vi "TestRUSH.vi"() -> ()   [LabVIEW 2012]
panel:
  out "Time in s":i32
  out "HavSetElevOut":i32
  in  "OutRoll":bool
  in  "Inroll":bool
  in  "Button 4":bool
  in  "Button 3":bool
  in  "Button 2":bool
  in  "Button1":bool
  out "HarvOutRollerB":dbl
  out "HarvOutRollerF":dbl
  out "HarvShootEnable":bool
  out "HarvOutElev":dbl
  in  "HarvClustIn":T1 {"HarvPOTElev" scale=0.0..5.0; "HarvManualElev" scale=-1.0..1.0; "HarvRollerBDesSpd" scale=-1.0..1.0; "HarvRollerFDesSpd" scale=-1.0..1.0}
  in  "LowerLimit":bool
  in  "UpperLimit":bool
  in  "HarvPOTElev":dbl(knob) scale=0.0..5.0
  in  "HarvManualElev":dbl(slide) scale=-1.0..1.0
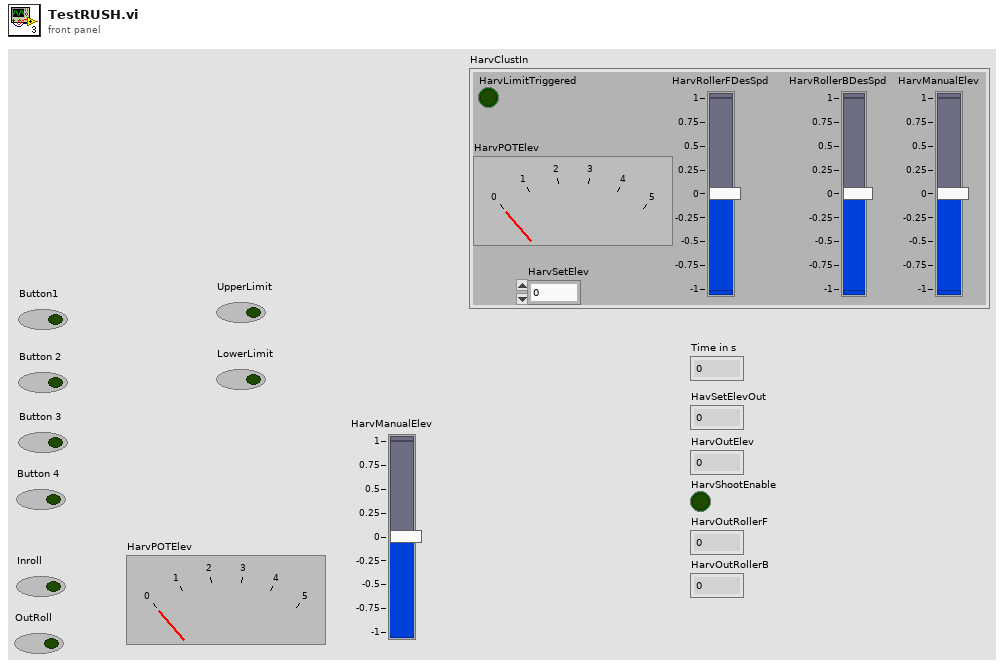
[diagram p1: front panel]
types:
  T1 = cluster{"HarvLimitTriggered":bool, "HarvRollerFDesSpd":dbl, "HarvRollerBDesSpd":dbl, "HarvManualElev":dbl, "HarvPOTElev":dbl, "HarvSetElev":i32}
  T2 = cluster{"HarvOutElev":dbl, "HarvShootEnable":bool, "HarvOutRollerF":dbl, "HarvOutRollerB":dbl, "HavSetElevOut":i32}
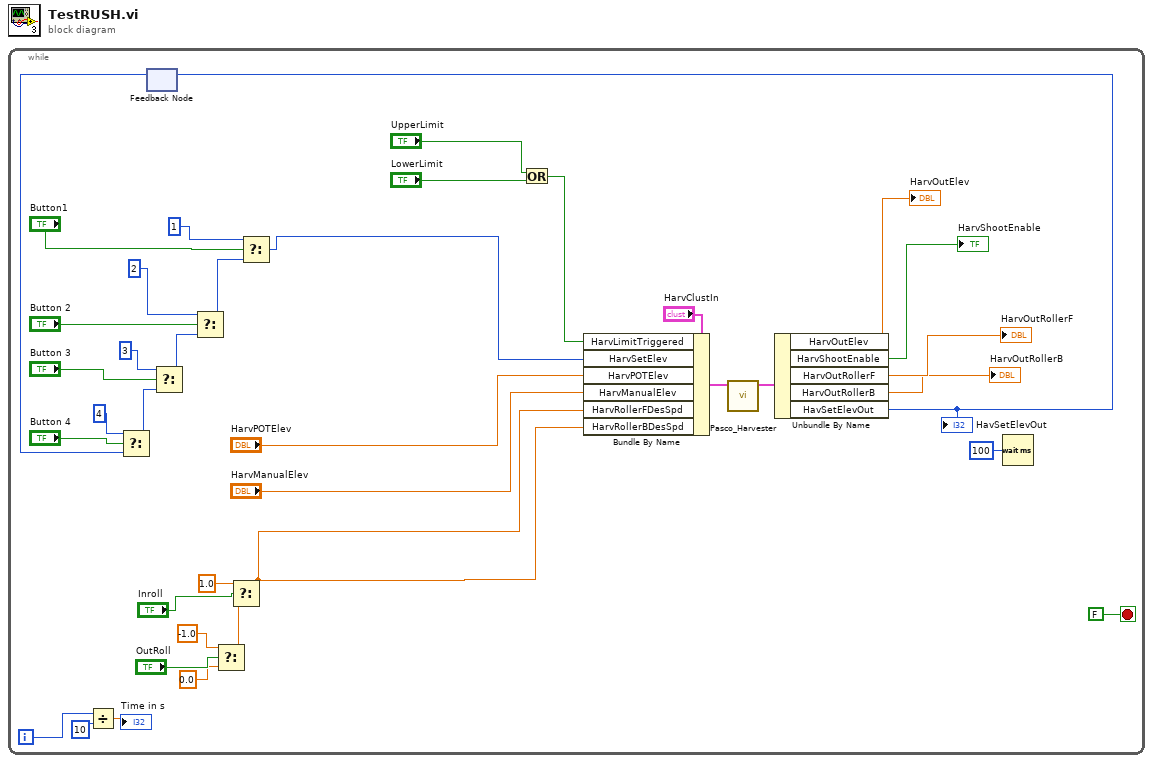
[diagram p0: block diagram]
diagram:
  n1 = while {
    i -> [w2]
    stop <- FALSE stop-if-true
    n2 = Divide(x=w2, y=10) -> (x/y=→"Time in s":dbl)
    n3 = feedback #1() -> (w5:i32)  [unwired: 1 in]
    n4 = Select(t=4, s="Button 4", f=w5) -> (s? t:f=w18:i32)
    n5 = Select(t=3, s="Button 3", f=w18) -> (s? t:f=w19:i32)
    n6 = Select(t=2, s="Button 2", f=w19) -> (s? t:f=w21:i32)
    n7 = Select(t=-1.0, s="OutRoll", f=0.0) -> (s? t:f=w8:dbl)
    n8 = Select(t=1.0, s="Inroll", f=w8) -> (s? t:f=w7:dbl)
    n9 = Select(t=1, s="Button1", f=w21) -> (s? t:f=w6:i32)
    n10 = Or(x="UpperLimit", y="LowerLimit") -> (x .or. y?=w31:bool)
    n11 = Bundle By Name(cluster="HarvClustIn", "HarvLimitTriggered"=w31, "HarvSetElev"=w6, "HarvPOTElev"="HarvPOTElev", "HarvManualElev"="HarvManualElev", "HarvRollerFDesSpd"=w7, "HarvRollerBDesSpd"=w7) -> (w32:T1)
    n12 = call "Pasco_Harvester.vi"("HarvClustIn"=w32) -> ("HarvClustOut"=w36:T2)  [unwired: 10 in]
    n13 = Unbundle By Name(w36) -> ("HarvOutElev"=→"HarvOutElev":dbl, "HarvShootEnable"=→"HarvShootEnable":bool, "HarvOutRollerF"=→"HarvOutRollerF":dbl, "HarvOutRollerB"=→"HarvOutRollerB":dbl, "HavSetElevOut"=w4:i32)
    "HavSetElevOut" <- w4
    n14 = feedback-in #1(w4) -> ()
    n15 = Wait (ms)(milliseconds to wait=u32 100) -> ()  [unwired: 1 out]
  }
